vi "Get MeasurementService Measure Request.vi"(8 "error in (no error)":errorcluster, 11 "gRPCid":T1) -> (0 "error out":errorcluster, 2 "Message Data":T2, 3 "gRPCid out":T1)   [LabVIEW 2020, in "Measurement Plugin Measurement Service Base V2.lvlib" / "MeasurementServiceBaseV2.lvclass"]
uses:
  MeasurementServiceBaseV2.lvclass
  RPC Messages/ni_measurementlink_measurement_v2_MeasureRequest.ctl
  RPC Messages/google_protobuf_Any.ctl
  RPC Messages/ni_measurementlink_PinMapContext.ctl
  <vilib>/gRPC/LabVIEW gRPC Library/Shared/grpcId.ctl
  Measurement Plugin Measurement Service Base V2.lvlib
  <vilib>/gRPC/LabVIEW gRPC Library/grpc-lvsupport-release.lvlib
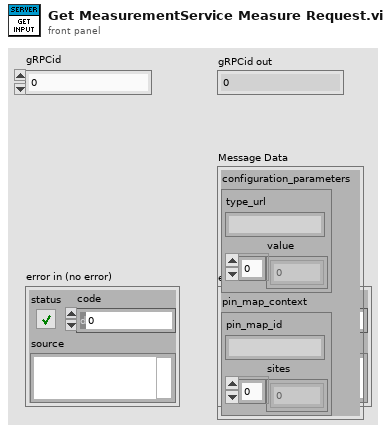
[diagram p1: front panel]
types:
  T1 = typedef "grpc-lvsupport-release.lvlib/grpcId.ctl" = u64
  T2 = typedef "Measurement Plugin Measurement Service Base V2.lvlib/ni_measurementlink_measurement_v2_MeasureRequest.ctl" = cluster{"configuration_parameters":T3, "pin_map_context":T4}
  T3 = typedef "Measurement Plugin Measurement Service Base V2.lvlib/google_protobuf_Any.ctl" = cluster{"type_url":string, "value":u8[]}
  T4 = typedef "Measurement Plugin Measurement Service Base V2.lvlib/ni_measurementlink_PinMapContext.ctl" = cluster{"pin_map_id":string, "sites":i32[]}
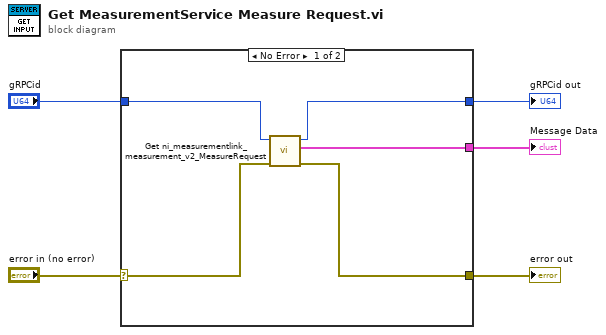
[diagram p0: block diagram]
diagram:
  n1 = case shown="No Error" "error in (no error)" {
    selector: "error in (no error)" -> [w10 w12]
    tunnel: [w9 w12] -> w4
    tunnel: [w8 _] -> w3
    tunnel: "gRPCid" -> [w7 w11]
    tunnel: [w6 w11] -> w1
    frame No Error {
      n2 = call "Get ni_measurementlink_measurement_v2_MeasureRequest.vi"("error in (no error)"=w10, "gRPCid"=w7) -> ("error out"=w9:errorcluster, "package_templatemessage"=w8:T2, "gRPCid out"=w6:T1)  [unwired: 7 in]
    }
    frame Error {
    }
  }
  "error out" <- w4
  "Message Data" <- w3
  "gRPCid out" <- w1
